vi "move_tilt_stage(Sub VI).vi"(0 "Axis inputs":T1={"Relative Steps"=0, "Motor Number"=1, "Run?"=FALSE, "Filename"=path "position.lvm", "CmdLib In"=refnum, "Device Address In"=0, "DeviceKey In"=""}, 1 "stop":bool, 2 "error in (no error)":errorcluster) -> (3 "CmdLib Out":refnum<k24>, 4 "DeviceKey Out":string, 5 "Position Status":i32, 6 "error out":errorcluster)   [LabVIEW 2016]
uses:
  C:/Users/UsphereLab/Documents/GitHub/Optlev/LabView Code/Tilt Stage/CmdLib.dll
  Tilt Stage/CmdLib.dll
panel:
  out "Description":string
  out "EOF?":bool
  out "Saving Data":bool
  out "Filename Out":path
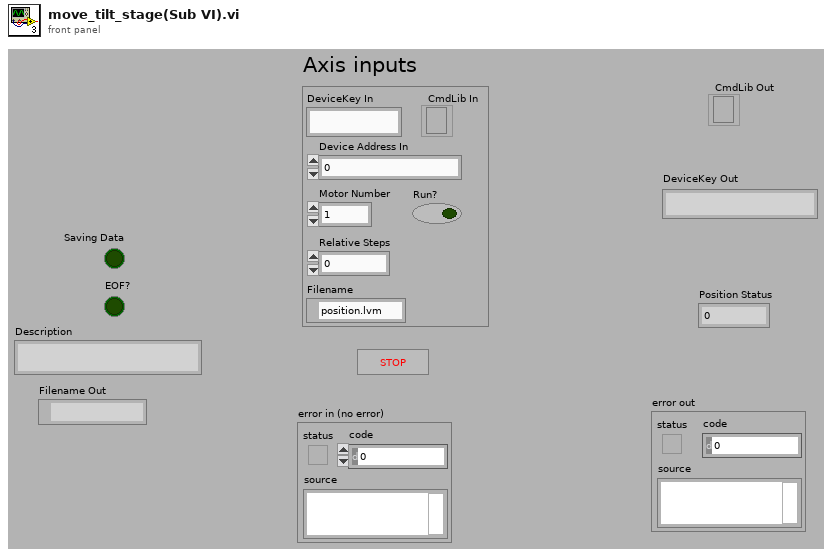
[diagram p1: front panel]
types:
  T1 = cluster{"Relative Steps":i32, "Motor Number":i32, "Run?":bool, "Filename":path, "CmdLib In":refnum<k24>, "Device Address In":i32, "DeviceKey In":string}
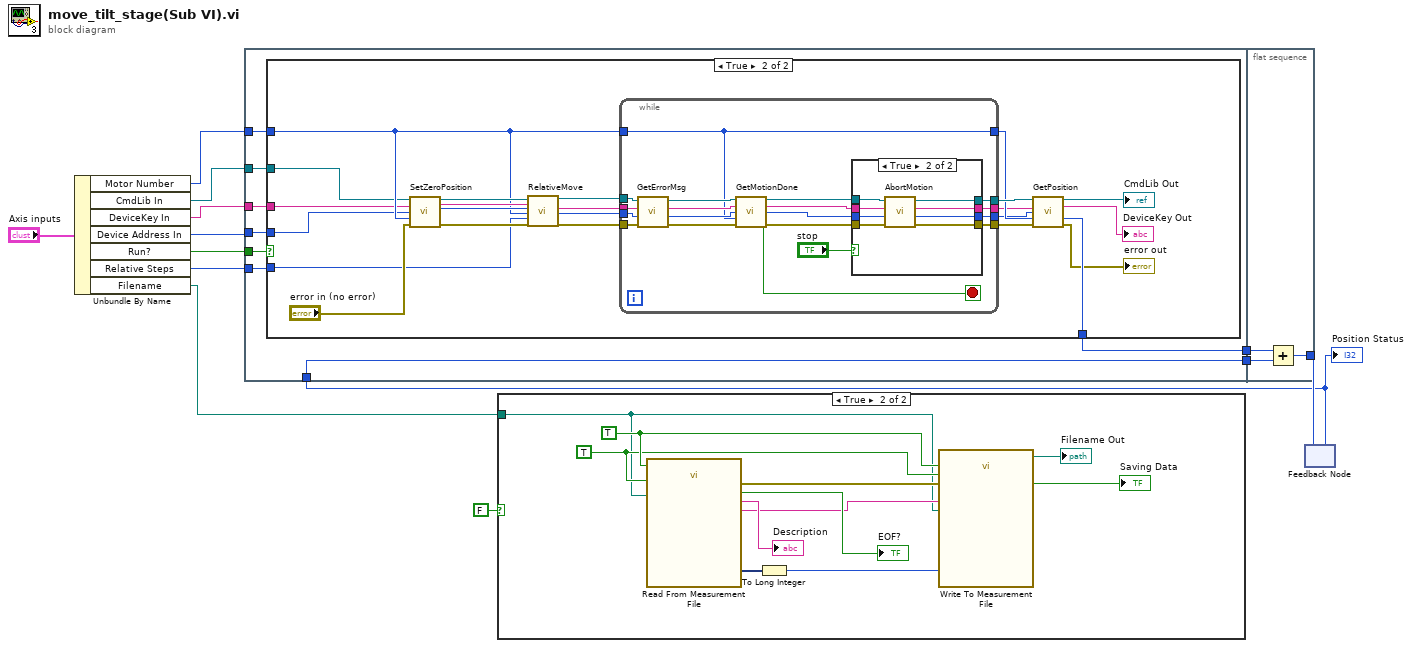
[diagram p0: block diagram]
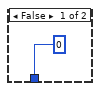
[diagram p3: hidden frame]
diagram:
  n1 = Unbundle By Name("Axis inputs") -> ("Motor Number"=w10:i32, "CmdLib In"=w9:refnum<k24>, "DeviceKey In"=w8:string, "Device Address In"=w7:i32, "Run?"=w6:bool, "Relative Steps"=w5:i32, "Filename"=w4:path)
  n2 = flat-sequence {
    tunnel: [w20] -> w13
    tunnel: w1 -> [w21]
    tunnel: [w21] -> w12
    tunnel: w10 -> [w19]
    tunnel: w9 -> [w18]
    tunnel: w8 -> [w17]
    tunnel: w7 -> [w16]
    tunnel: w6 -> [w15]
    tunnel: w5 -> [w14]
    tunnel: [w77] -> w2
    tunnel: w13 -> [w78]
    tunnel: w12 -> [w79]
    frame #0 {
      n3 = case shown="True" w15 {
        tunnel: [0 ("Relative Steps") w32] -> w20
        tunnel: w19 -> [_ w30]
        tunnel: w18 -> [_ w29]
        tunnel: w17 -> [_ w28]
        tunnel: w16 -> [_ w27]
        tunnel: w14 -> [_ w26]
        frame False {
        }
        frame True {
          n4 = call "SetZeroPosition.vi"("CmdLib In"=w29, "DeviceKey In"=w28, "Device Address In"=w27, "Motor"=w30, "error in (no error)"="error in (no error)") -> ("CmdLib Out"=w42:refnum<k24>, "DeviceKey Out"=w41:string, "Device Address Out"=w39:i32, "error out"=w40:errorcluster)  [unwired: 7 in]
          n5 = call "RelativeMove.vi"("CmdLib In"=w42, "DeviceKey In"=w41, "Device Address In"=w39, "Motor"=w30, "Relative Steps"=w26, "error in (no error)"=w40) -> ("CmdLib Out"=w45:refnum<k24>, "DeviceKey Out"=w44:string, "Device Address Out"=w38:i32, "error out"=w43:errorcluster)  [unwired: 10 in]
          n6 = while {
            tunnel: w30 -> [w49]
            tunnel: w45 -> [w62]
            tunnel: w44 -> [w61]
            tunnel: [w57] -> w36
            tunnel: w38 -> [w56]
            tunnel: w43 -> [w60]
            tunnel: [w58] -> w37
            tunnel: [w49] -> w35
            tunnel: [w48] -> w34
            tunnel: [w47] -> w33
            stop <- w54 stop-if-true
            n7 = call "GetErrorMsg.vi"("error in (no error)"=w60, "Device Address In"=w56, "DeviceKey In"=w61, "CmdLib In"=w62) -> ("error out"=w59:errorcluster, "Device Address Out"=w55:i32, "DeviceKey Out"=w64:string, "CmdLib Out"=w63:refnum<k24>)
            n8 = call "GetMotionDone.vi"("CmdLib In"=w63, "DeviceKey In"=w64, "Device Address In"=w55, "Motor"=w49, "error in (no error)"=w59) -> ("CmdLib Out"=w53:refnum<k24>, "DeviceKey Out"=w52:string, "Device Address Out"=w51:i32, "Is Motion Done"=w54:bool, "error out"=w50:errorcluster)  [unwired: 6 in]
            n9 = case shown="True" "stop" {
              tunnel: w50 -> [w67 w76]
              tunnel: [w67 w75] -> w58
              tunnel: w53 -> [w68 w74]
              tunnel: [w68 w73] -> w57
              tunnel: w52 -> [w65 w72]
              tunnel: w51 -> [w66 w71]
              tunnel: [w66 w70] -> w48
              tunnel: [w65 w69] -> w47
              frame False {
              }
              frame True {
                n10 = call "AbortMotion.vi"("error in (no error)"=w76, "Device Address In"=w71, "DeviceKey In"=w72, "CmdLib In"=w74) -> ("error out"=w75:errorcluster, "Device Address Out"=w70:i32, "DeviceKey Out"=w69:string, "CmdLib Out"=w73:refnum<k24>)
              }
            }
          }
          n11 = call "GetPosition.vi"("CmdLib In"=w36, "DeviceKey In"=w33, "Device Address In"=w34, "Motor"=w35, "error in (no error)"=w37) -> ("CmdLib Out"=→"CmdLib Out":refnum<k24>, "DeviceKey Out"=→"DeviceKey Out":string, "Position"=w32:i32, "error out"=→"error out":errorcluster)  [unwired: 6 in, 1 out]
        }
      }
    }
    frame #1 {
      n12 = Add(x=w78, y=w79) -> (x+y=w77:i32)
    }
  }
  n13 = case shown="True" FALSE {
    tunnel: w4 -> [_ w81]
    frame False {
    }
    frame True {
      w83 = TRUE ("Enable")
      w84 = TRUE ("Reset")
      n14 = call "Read From Measurement File"("Filename"=w81, "Enable"=w83, "Reset"=w84) -> ("error out"=w86:errorcluster, "Signals"=w82:dynamicdata, "EOF?"=→"EOF?":bool, "Comment"=w85:string, "Description"=→"Description":string)  [unwired: 3 in, 1 out]
      n15 = To Long Integer(number=w82) -> (32bit integer=w80:i32)
      n16 = call "Write To Measurement File"("Signals"=w80, "Reset"=w84, "Enable"=w83, "error in (no error)"=w86, "Filename"=w81, "Comment"=w85) -> ("Filename Out"=→"Filename Out":path, "Saving Data"=→"Saving Data":bool)  [unwired: 11 in, 1 out]
    }
  }
  n17 = feedback-in #1(w2) -> ()
  n18 = feedback #1() -> (w1:i32)  [unwired: 1 in]
  "Position Status" <- w1
